vi "Update Enum Entries.vi"(4 "Enumeration":T2, 6 "Built Enumeration":T1, 7 "App":refnum<vi>, 8 "error in (no error)":errorcluster, 11 "LV-Protoc in":refnum<class "LV-Protoc.lvclass">) -> (0 "error out":errorcluster, 2 "Values":i32[](array[numeric]), 3 "LV-Protoc out":refnum<class "LV-Protoc.lvclass">)   [LabVIEW 2020, in "LV-Protoc.lvlib" / "LV-Protoc.lvclass"]
uses:
  LV-Protoc.lvclass
  LV-Proto/Enumeration.ctl
  LV-Proto/Enum Value.ctl
  Enumeration Paths.ctl
  b5b19fd3-6fd5-4925-8503-100cde87289d.vi
  <vilib>/Comparison/Less/Less Functor/Less Functor.lvclass
  LV-Protoc.lvlib
  LV-Proto/LV-Proto.lvlib
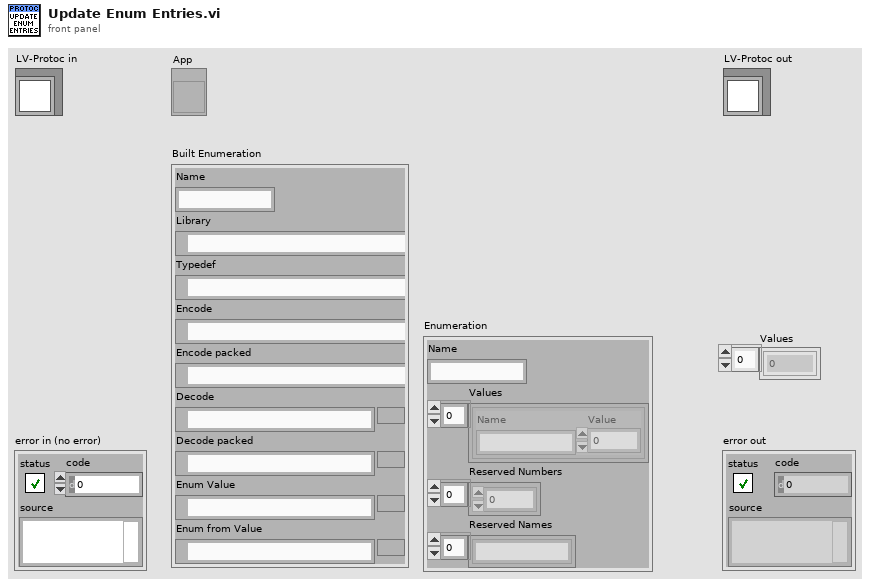
[diagram p1: front panel]
types:
  T1 = typedef "LV-Protoc.lvlib/Enumeration Paths.ctl" = cluster{"Name":string, "Library":path, "Typedef":path, "Encode":path, "Encode packed":path, "Decode":path, "Decode packed":path, "Enum Value":path, "Enum from Value":path}
  T2 = typedef "LV-Proto.lvlib/Enumeration.ctl" = cluster{"Name":string, "Values":T3[], "Reserved Numbers":u32[], "Reserved Names":string[]}
  T3 = typedef "LV-Proto.lvlib/Enum Value.ctl" = cluster{"Name":string, "Value":i32}
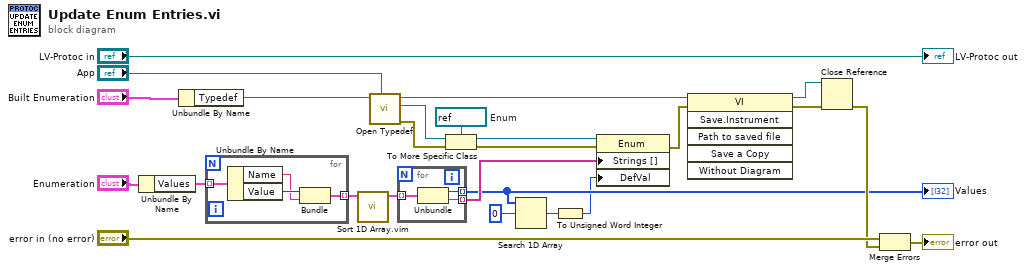
[diagram p0: block diagram]
diagram:
  w25 = refnum<vi> refnum  # Enum
  n1 = Unbundle By Name("Enumeration") -> ("Values"=w21:T3[])
  n2 = Unbundle By Name("Built Enumeration") -> ("Typedef"=w12:path)
  n3 = for {
    tunnel: w21 -> [w29] mode=indexing
    tunnel: [w26] -> w16 mode=indexing
    n4 = Unbundle By Name(w29) -> ("Name"=w27:string, "Value"=w28:i32)
    n5 = Bundle("Value"=w28, "Name"=w27) -> (w26:cluster{"Value":i32, "Name":string})  [unwired: 1 in]
  }
  n6 = call "Sort 1D Array.vim"("unsorted array"=w16) -> ("sorted array"=w15:cluster{"Value":i32, "Name":string}[])  [unwired: 10 in]
  n7 = call "Open Typedef.vi"("App"="App", "Typedef Path"=w12) -> ("error out"=w7:errorcluster, "Control"=w10:refnum<vi>, "VI"=w11:refnum<vi>)  [unwired: 7 in]
  n8 = for {
    tunnel: w15 -> [w32] mode=indexing
    tunnel: [w31] -> w14 mode=indexing
    tunnel: [w30] -> w4 mode=indexing
    n9 = Unbundle(w32) -> ("Value"=w30:i32, "Name"=w31:string)
  }
  "Values" <- w4
  n10 = To More Specific Class(target class=w25, reference=w10, error in=w7) -> (specific class reference=w24:refnum<vi>, error out=w23:errorcluster)
  n11 = Search 1D Array(1D array=w4, element=0) -> (index of element=w2:i32)  [unwired: 1 in]
  n12 = To Unsigned Word Integer(number=w2) -> (unsigned 16bit integer=w1:u16)
  n13 = property class="Enum"(reference=w24, error in=w23, "Strings []"=w14, "DefVal"=w1) -> (error out=w18:errorcluster)  [unwired: 1 out]
  n14 = invoke class="VI" method="Save.Instrument"(reference=w11, error in=w18) -> (reference out=w8:refnum<vi>, error out=w9:errorcluster)  [unwired: 4 in, 4 out]
  n15 = Close Reference(reference=w8, error in (no error)=w9) -> (error out=w6:errorcluster)
  n16 = Merge Errors("error in (no error)", w6) -> (→"error out":errorcluster)
  "LV-Protoc out" <- "LV-Protoc in"
